vi "Cast Object to Variant.vi"(8 "error in (no error)":errorcluster, 9 "datatype and defaults":variant, 11 "JSON Value in":refnum<class "JSON Value.lvclass">) -> (0 "error out":errorcluster, 1 "defaulted keys":string[](array[string]), 2 "Variant":variant)   [LabVIEW 2016, in "JSON Value.lvclass"]
doc: "Populates a variant with the data contained in the given JSON instance. Valid types for datatype and defaults are: string, boolean, double, and a cluster of named controls of strings, booleans, doubles, or nested clusters.\n\nIf a given cluster contains values that aren't present in the JSON Object instance, the value in the datatype and defaults control is used instead and the defaulted keys output will contain the name of the path in the cluster to the control."
uses:
  JSON Value.lvclass
  Object/Get Value/Get Value (JSON).vi
  <vilib>/Utility/Data Type/NI_Data Type.lvlib
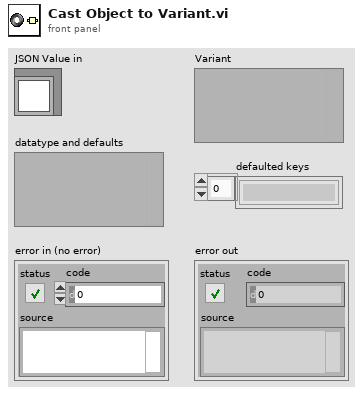
[diagram p1: front panel]
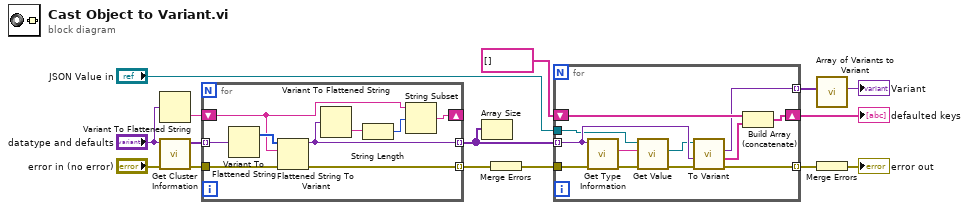
[diagram p0: block diagram]
diagram:
  n1 = Variant To Flattened String(Variant="datatype and defaults") -> (data string=w11:string)  [unwired: 1 out]
  n2 = call <vilib>:"Get Cluster Information.vi"("error in (no error)"="error in (no error)", "Variant"="datatype and defaults") -> ("error out"=w9:errorcluster, "Cluster Elements"=w10:variant[])  [unwired: 8 in]
  n3 = for {
    tunnel: w10 -> [w24] mode=indexing
    tunnel: [w22] -> w6 mode=indexing
    shift-right: [w18] -> _
    shift-left: w11 -> [w21]
    tunnel: w9 -> [w17]
    tunnel: [w16] -> w4 mode=indexing
    n4 = Variant To Flattened String(Variant=w24) -> (1:w23:i16[])  [unwired: 1 out]
    n5 = Flattened String To Variant(4:w17, 6:w21, 7:w23) -> (0:w16:errorcluster, 3:w22:variant)
    n6 = Variant To Flattened String(Variant=w22) -> (data string=w20:string)  [unwired: 1 out]
    n7 = String Length(string=w20) -> (length=w19:i32)
    n8 = String Subset(string=w21, offset (0)=w19) -> (substring=w18:string)  [unwired: 1 in]
  }
  n9 = Array Size(array=w6) -> ()  [unwired: 1 out]
  n10 = Merge Errors(w4) -> (w5:errorcluster)
  n11 = for {
    tunnel: w6 -> [w36] mode=indexing
    tunnel: "JSON Value in" -> [w35]
    tunnel: [w34] -> w13 mode=indexing
    tunnel: w5 -> [w33]
    shift-right: [w31] -> w2
    shift-left: string[] [] -> [w32]
    tunnel: [w30] -> w1 mode=indexing
    n12 = call <vilib>:"Get Type Information.vi"("error in (no error)"=w33, "Variant"=w36) -> ("error out"=w26:errorcluster, "Name"=w28:string)  [unwired: 5 in, 3 out]
    n13 = call-poly "Get Value.vi"("error in (no error)"=w26, "key"=w28, "JSON Value in"=w35) -> ("error out"=w25:errorcluster, "JSON Value out"=w27:refnum<class "JSON Value.lvclass">)  [unwired: 7 in]
    n14 = call "To Variant.vi"("error in (no error)"=w25, "datatype and defaults"=w36, "JSON Value in"=w27) -> ("error out"=w34:errorcluster, "defaulted keys"=w29:string[], "Variant"=w30:variant)  [unwired: 6 in]
    n15 = Build Array (concatenate)(w32, w29) -> (w31:string[])
  }
  "defaulted keys" <- w2
  n16 = call "Array of Variants to Variant.vi"("Array"=w1) -> ("Variant"=→"Variant":variant)  [unwired: 10 in]
  n17 = Merge Errors(w13) -> (→"error out":errorcluster)
